vi "Sensors Data.vi"(7 "Read//Write":T1, 8 "Distance In":dbl, 9 "Switch Hit?":bool, 10 "Limit Down In":bool, 11 "Limit Up In":bool) -> (0 "Distance Out":dbl, 1 "Switch Hit Out":bool, 2 "Limit Down Out":bool, 3 "Limit Up Out":bool)   [LabVIEW 2018]
uses:
  Type Defs/Read Write.ctl
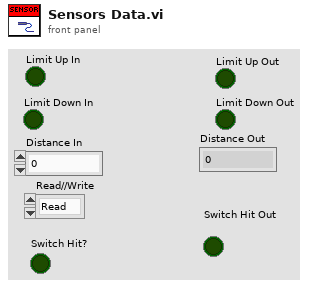
[diagram p1: front panel]
types:
  T1 = typedef "Read Write.ctl" = enum16{"Read", "Write"}
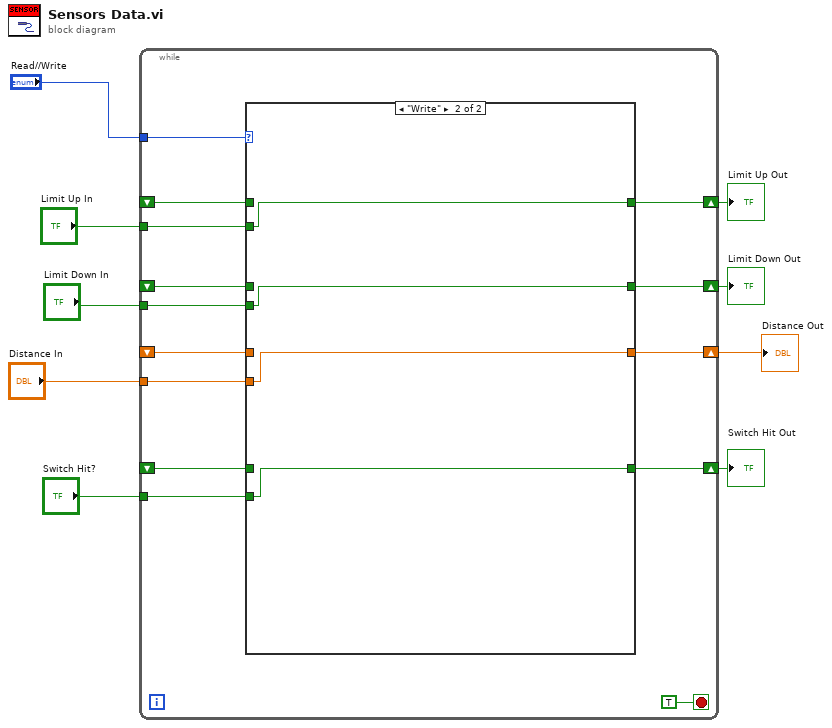
[diagram p0: block diagram]
diagram:
  n1 = while {
    tunnel: "Read//Write" -> [w22]
    shift-right: [w21] -> w8
    shift-left: _ -> [w19]
    shift-right: [w20] -> w7
    shift-left: _ -> [w18]
    tunnel: "Limit Up In" -> [w17]
    tunnel: "Limit Down In" -> [w16]
    shift-right: [w14] -> w4
    shift-left: _ -> [w13]
    tunnel: "Distance In" -> [w15]
    tunnel: "Switch Hit?" -> [w12]
    shift-right: [w10] -> w1
    shift-left: _ -> [w11]
    stop <- TRUE stop-if-true
    n2 = case shown="\"Write\"" w22 {
      tunnel: [w27 w31] -> w21
      tunnel: [w26 w30] -> w20
      tunnel: w19 -> [w27 _]
      tunnel: w18 -> [w26 _]
      tunnel: w17 -> [_ w31]
      tunnel: w16 -> [_ w30]
      tunnel: w15 -> [_ w29]
      tunnel: [w25 w29] -> w14
      tunnel: w13 -> [w25 _]
      tunnel: w12 -> [_ w28]
      tunnel: w11 -> [w24 _]
      tunnel: [w24 w28] -> w10
      frame "Read", Default {
      }
      frame "Write" {
      }
    }
  }
  "Limit Up Out" <- w8
  "Limit Down Out" <- w7
  "Distance Out" <- w4
  "Switch Hit Out" <- w1
